vi "proyecto.vi"() -> ()   [LabVIEW 2010]
uses:
  <vilib>/Daq/1easyio.llb/AI Acquire Waveform (waveform).vi
panel:
  in  "device":i16=1
  out "Waveform Chart":dbl(graph)
  in  "Presion baja":bool
  in  "Histeresis":dbl
  in  "Umbral":dbl
  out "COMPRESOR ON":bool
  in  "ENCENDIDO DEL SISTEMA":bool
  # "ON"
  # "OFF"
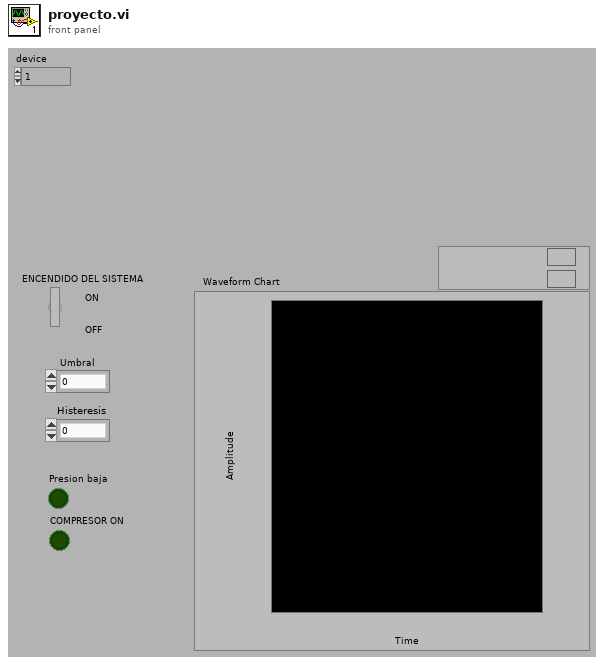
[diagram p1: front panel]
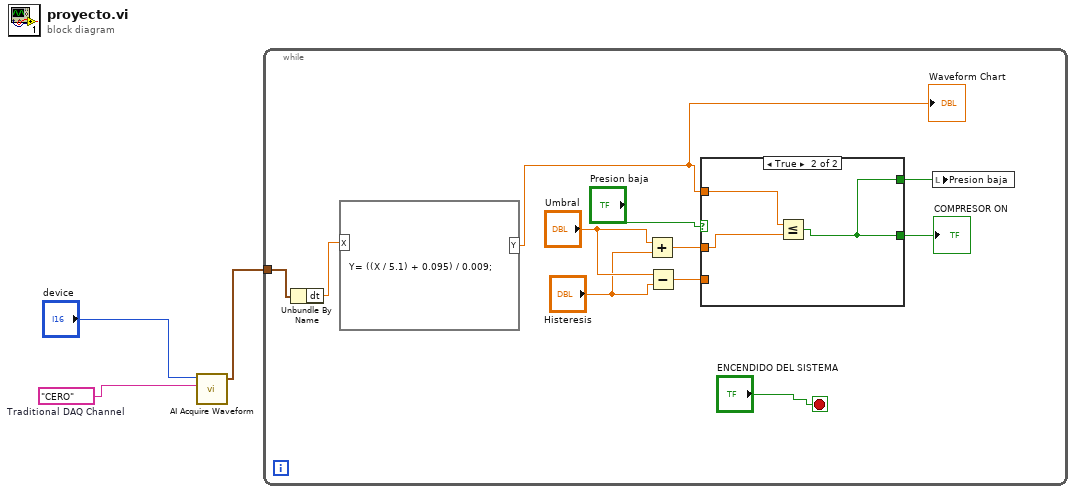
[diagram p0: block diagram]
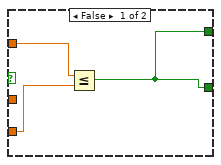
[diagram p2: hidden frame]
diagram:
  w1 = tag "CERO"  # Traditional DAQ Channel
  n1 = call-poly <vilib>:"AI Acquire Waveform.vi"("channel (0)"=w1, "device"="device") -> ("waveform"=w2:waveform(dbl))  [unwired: 6 in]
  n2 = while {
    tunnel: w2 -> [w6]
    stop <- "ENCENDIDO DEL SISTEMA" stop-if-true
    n3 = Unbundle By Name(w6) -> ("dt"=w5:dbl)
    n4 = formula code="Y= ((X / 5.1) + 0.095) / 0.009;"("X"=w5) -> ("Y"=w4:dbl)
    "Waveform Chart" <- w4
    n5 = Add(x="Umbral", y="Histeresis") -> (x+y=w10:dbl)
    n6 = Subtract(x="Umbral", y="Histeresis") -> (x-y=w11:dbl)
    n7 = case shown="True" "Presion baja" {
      tunnel: [w15 w18] -> w13
      tunnel: [w15 w18] -> w12
      tunnel: w11 -> [w17 _]
      tunnel: w10 -> [_ w19]
      tunnel: w4 -> [w16 w20]
      frame False {
        n8 = Less Or Equal?(x=w16, y=w17) -> (x <= y?=w15:bool)
      }
      frame True {
        n9 = Less Or Equal?(x=w20, y=w19) -> (x <= y?=w18:bool)
      }
    }
    "COMPRESOR ON" <- w12
    n10 = local write "Presion baja"(w13) -> ()
  }
